vi "PCT_Ranges.vi"(7 "mode":u8, 9 "Raw":cluster{"Min":sgl, "Max":sgl}, 11 "Python in":string="import machine, utime\n\ntx = machine.Pin('Y9', machine.Pin.OUT)\nrx = machine.Pin('Y10', machine.Pin.IN)\ntx.value(b'\\x00')\nutime.sleep_ms(500)\ntx.value(1)\n\nuart = machine.UART(3)\nuart.init(baudrate=2400, bits=8, parity=None, stop=1)\n\nuart.write(0)\nuart.write(b'\\x40\\x23\\x9C')\nuart.write(b'\\x98\\x00\\x4C\\x69\\x67\\x68\\x74\\x00\\x00\\x00\\x39')\n") -> (3 "Python out":string="import machine, utime\n\ntx = machine.Pin('Y9', machine.Pin.OUT)\nrx = machine.Pin('Y10', machine.Pin.IN)\ntx.value(b'\\x00')\nutime.sleep_ms(500)\ntx.value(1)\n\nuart = machine.UART(3)\nuart.init(baudrate=2400, bits=8, parity=None, stop=1)\n\nuart.write(0)\nuart.write(b'\\x40\\x23\\x9C')\nuart.write(b'\\x98\\x00\\x4C\\x69\\x67\\x68\\x74\\x00\\x00\\x00\\x39')\nuart.write(b'\\x90\\x80\\x01\\x00\\x03\\x00\\xED')\n")   [LabVIEW 2016]
panel:
  out "data string":string
  out "bytes added":u8[](array[numeric])=[144, 128, 1, 0, 3, 0, 237] format="%.0x"
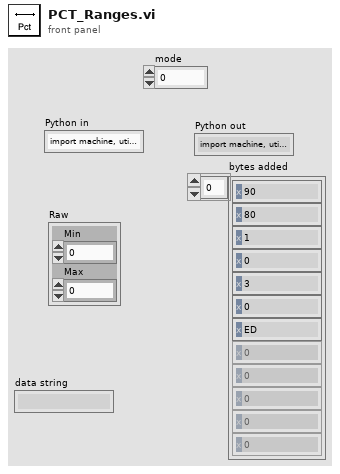
[diagram p1: front panel]
types:
  T1 = enum16{"big-endian, network order", "native, host order", "little-endian"}
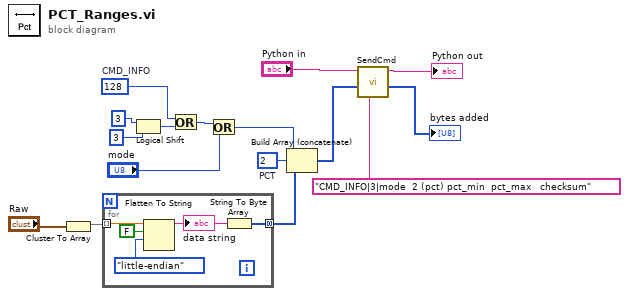
[diagram p0: block diagram]
diagram:
  w4 = u8 2  # PCT
  w12 = u8 128  # CMD_INFO
  n1 = Cluster To Array(cluster="Raw") -> (array=w3:sgl[])
  n2 = for {
    tunnel: w3 -> [w21] mode=indexing
    tunnel: [w17] -> w2 mode=concatenating
    n3 = Flatten To String(anything=w21, prepend array or string size? (T)=FALSE, byte order (0:big-endian, network order)=T1."little-endian") -> (data string=w19:string)  [unwired: 1 in, 2 out]
    "data string" <- w19
    n4 = String To Byte Array(string=w19) -> (unsigned byte array=w17:u8[])
  }
  n5 = Logical Shift(y=i16 3, x=u8 3) -> (x << y=w11:u8)
  n6 = Or(x=w12, y=w11) -> (x .or. y?=w13:u8)
  n7 = Or(x=w13, y="mode") -> (x .or. y?=w5:u8)
  n8 = Build Array (concatenate)(w5, w4, w2) -> (w6:u8[])
  n9 = call "SendCmd.vi"("Comment"="CMD_INFO|3|mode  2 (pct) pct_min  pct_max   checksum", "Array In"=w6, "Python in"="Python in") -> ("Array Sent"=→"bytes added":u8[], "Python out"=→"Python out":string)  [unwired: 7 in]
